vi "timetest7.vi"() -> ()   [LabVIEW 2015]
uses:
  BERTTA.dll
panel:
  in  "pause":i32
  in  "ramp_elapsed":i32
  in  "direction":i32
  out "setpoint":dbl
  in  "enable":i32
  in  "Tinit":dbl
  in  "Tset":dbl
  in  "ramp_time":i32
  out "Waveform Chart":dynamicdata(graph)
  out "Current temp":dbl
  out "elapsed (float)":dbl
  out "elapsed (int)":i32
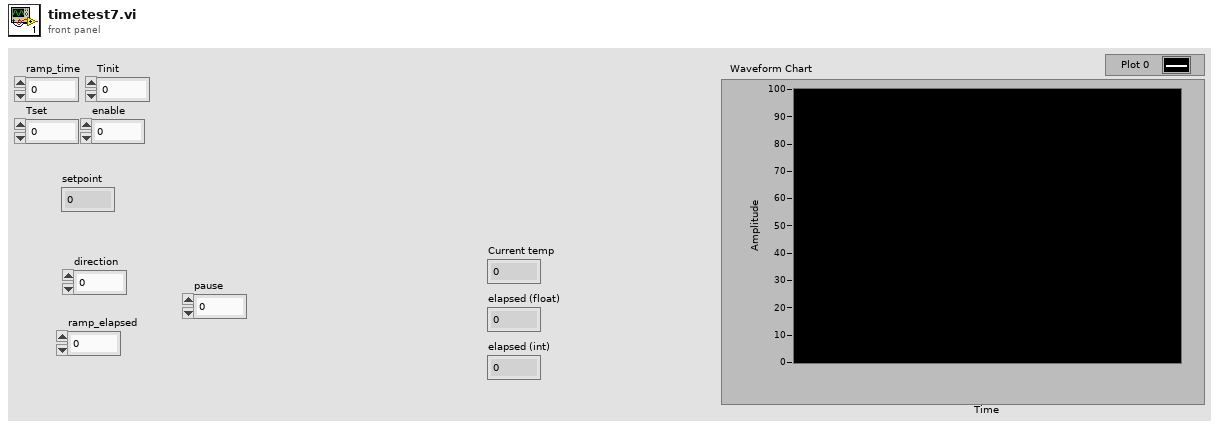
[diagram p1: front panel]
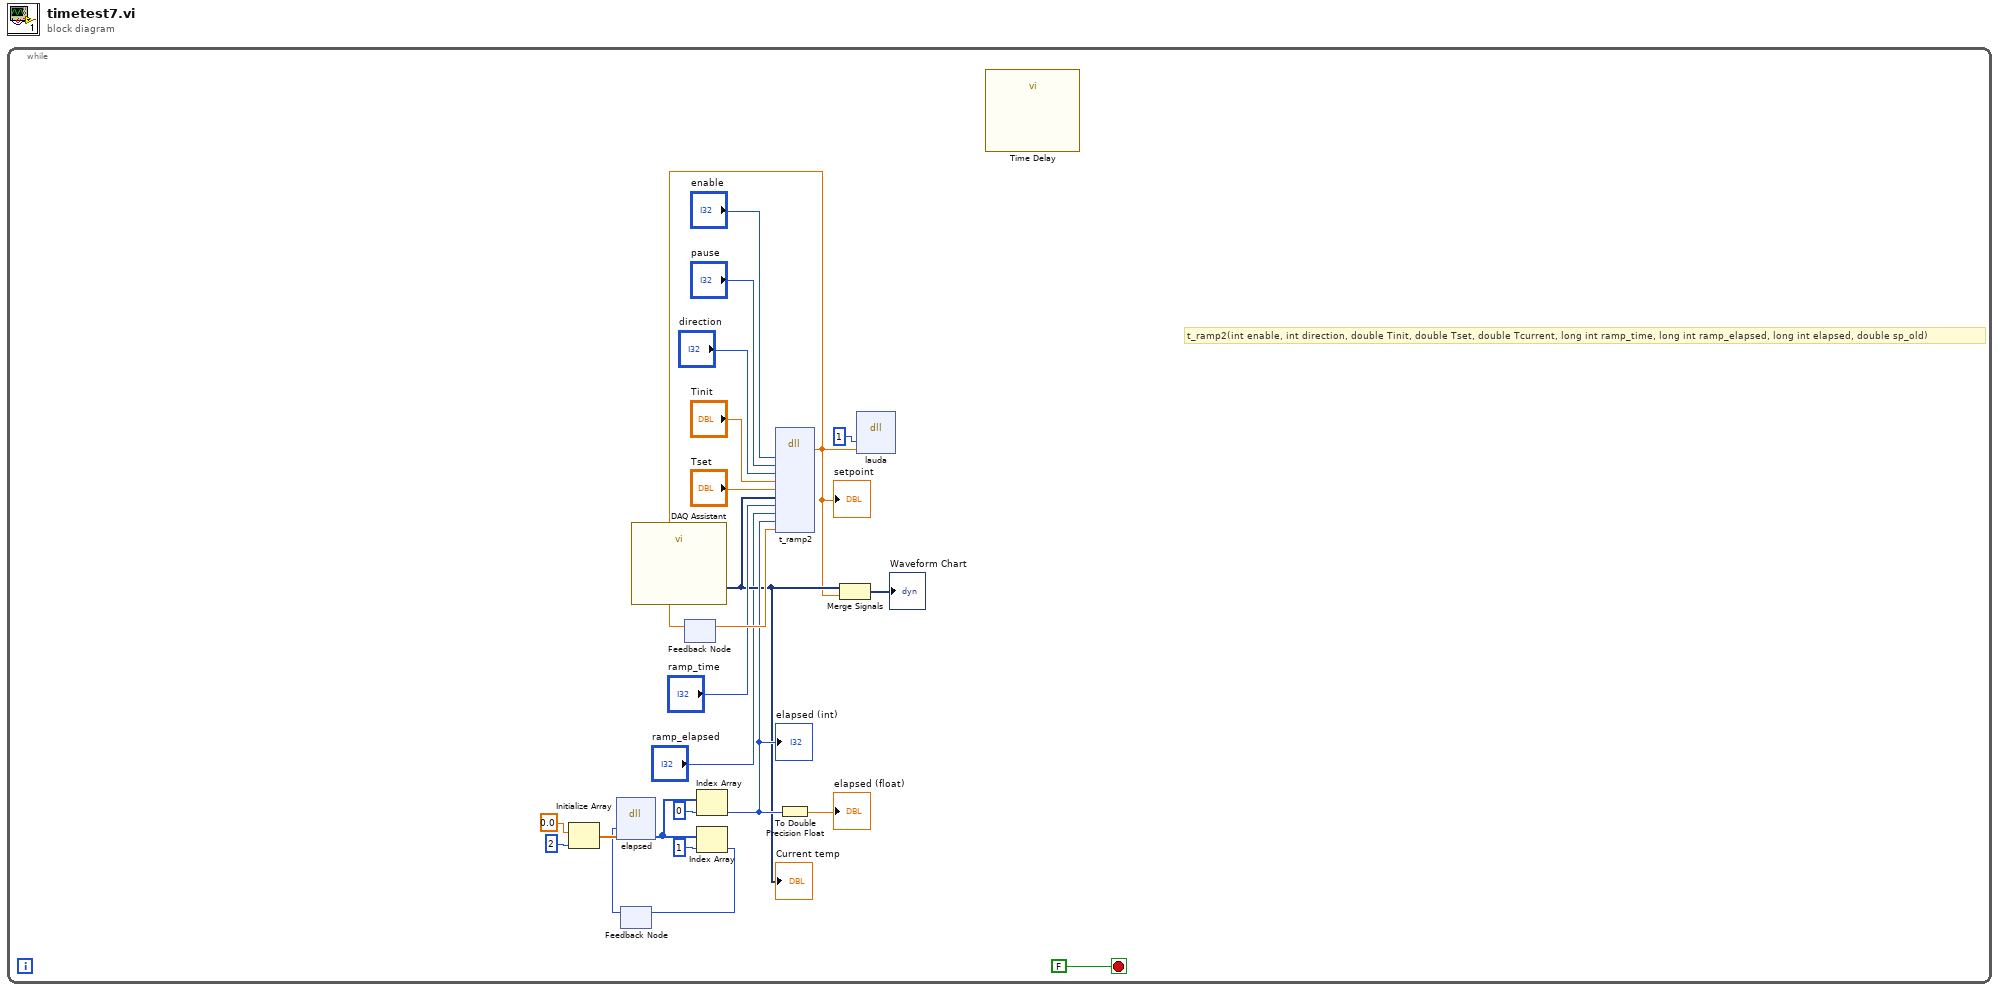
[diagram p0: block diagram]
diagram:
  n1 = while {
    stop <- FALSE stop-if-true
    # "t_ramp2(int enable, int direction, double Tinit, double Tset, double Tcurrent, long int ramp_time, long int ramp_elapsed, long int elapsed, double sp_old)"
    n2 = Initialize Array(0.0 ("element"), 2 ("dimension size")) -> (w23:dbl[])
    n3 = feedback #1() -> (w16:i32)  [unwired: 1 in]
    n4 = dll-call lib="C:/Users/xlaraser/Documents/Visual Studio 2017/Projects/Bertta/BERTTA/Debug/BERTTA.dll" fn="elapsed"("last_time"=w16, "params"=w23) -> ("params"=w19:i32[])  [unwired: 5 in, 2 out]
    n5 = call "DAQ Assistant"() -> ("data"=w8:dynamicdata)  [unwired: 17 in, 2 out]
    "Current temp" <- w8
    n6 = feedback #2() -> (w11:dbl)  [unwired: 1 in]
    n7 = Index Array(array=w19, index=0) -> (element=w10:i32)
    "elapsed (int)" <- w10
    n8 = Index Array(array=w19, index=1) -> (element=w17:i32)
    n9 = feedback-in #1(w17) -> ()
    n10 = dll-call lib="C:/Users/xlaraser/Documents/Visual Studio 2017/Projects/Bertta/BERTTA/Debug/BERTTA.dll" fn="t_ramp2"("enable"="enable", "pause"="pause", "direction"="direction", "Tinit"="Tinit", "Tset"="Tset", "Tcurrent"=w8, "ramp_time"="ramp_time", "ramp_elapsed"="ramp_elapsed", "elapsed"=w10, "sp_old"=w11) -> ("return type"=w4:dbl)  [unwired: 13 in, 2 out]
    "setpoint" <- w4
    n11 = feedback-in #2(w4) -> ()
    n12 = To Double Precision Float(number=w10) -> (double precision float=→"elapsed (float)":dbl)
    n13 = Merge Signals(w8, w4) -> (→"Waveform Chart":dynamicdata)
    n14 = dll-call lib="C:/Users/xlaraser/Documents/Visual Studio 2017/Projects/Bertta/BERTTA/Debug/BERTTA.dll" fn="lauda"("port"=1, "set_temp"=w4) -> ()  [unwired: 6 in, 2 out]
    n15 = call "Time Delay"() -> ()  [unwired: 11 in, 1 out]
  }
